vi "F Inverse CDF Array.vi"(8 "Error In":errorcluster, 9 "N2":i32, 10 "N1":i32, 11 "CDF(x) Array":dbl[](array[numeric])) -> (0 "Error Out":errorcluster, 3 "x Array":dbl[](array[numeric]))   [LabVIEW 2021, in "Math.lvlib"]
uses:
  <vilib>/gmath/statdist.llb/F Inverse CDF.vi
  Math.lvlib
  <vilib>/gmath/NI_Gmath.lvlib
  Error/Error.lvlib
  Time/Time.lvlib
panel:
  out "CPU (s)":dbl
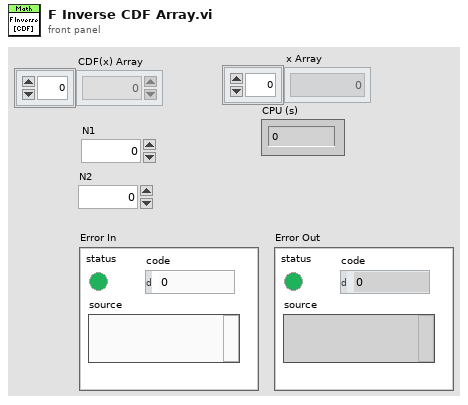
[diagram p1: front panel]
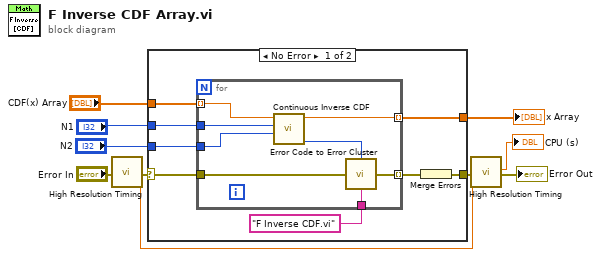
[diagram p0: block diagram]
diagram:
  n1 = call "High Resolution Timing.vi"("Error In"="Error In") -> ("elapsed (relative) seconds"=w2:dbl, "Error Out"=w4:errorcluster)  [unwired: 16 in, 1 out]
  n2 = case shown="No Error" w4 {
    selector: w4 -> [w14 w27]
    tunnel: "CDF(x) Array" -> [w18 _]
    tunnel: [w17 _] -> w9
    tunnel: "N1" -> [w16 _]
    tunnel: "N2" -> [w15 _]
    tunnel: [w12 w27] -> w5
    frame No Error {
      n3 = for {
        tunnel: w18 -> [w26] mode=indexing
        tunnel: w16 -> [w25]
        tunnel: [w24] -> w17 mode=indexing
        tunnel: w15 -> [w23]
        tunnel: [w21] -> w13 mode=indexing
        tunnel: w14 -> [w20]
        tunnel: "F Inverse CDF.vi" ("Error Source") -> [w19]
        n4 = call-poly <vilib>:"Continuous Inverse CDF.vi"("k2"=w23, "k1"=w25, "cdf(x)"=w26) -> ("error"=w22:i32, "x"=w24:dbl)  [unwired: 7 in]
        n5 = call "Error Code to Error Cluster.vi"("Error Code"=w22, "Error Source"=w19, "Error In"=w20) -> ("Error Out"=w21:errorcluster)  [unwired: 12 in]
      }
      n6 = Merge Errors(w13) -> (w12:errorcluster)
    }
    frame Error {
    }
  }
  "x Array" <- w9
  n7 = call "High Resolution Timing.vi"("relative seconds (NaN)"=w2, "Error In"=w5) -> ("elapsed (relative) seconds"=→"CPU (s)":dbl, "Error Out"=→"Error Out":errorcluster)  [unwired: 15 in, 1 out]
